vi "Práctica01_Ejercicio2_4.vi"() -> ()   [LabVIEW 2020]
panel:
  out "?":string
  in  "Selector de Operación":i16(knob) scale=0.0..3.0
  in  "y":dbl
  in  "x":dbl
  # "Resta"
  # "Multiplicacion"
  # "Division"
  # "Suma"
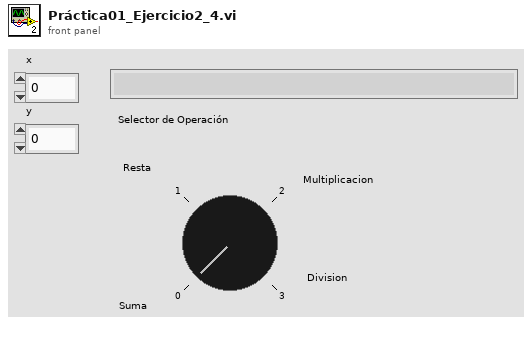
[diagram p1: front panel]
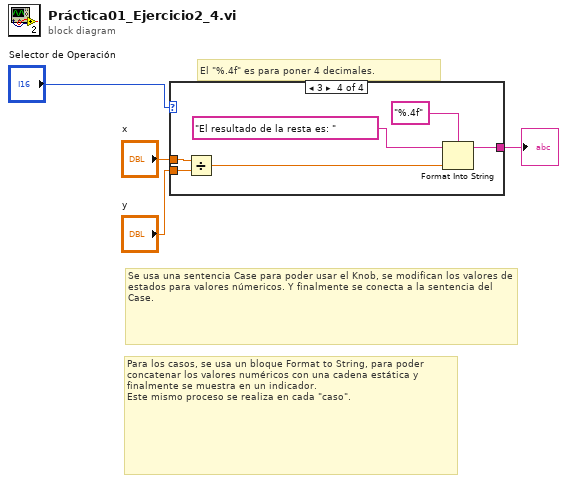
[diagram p0: block diagram]
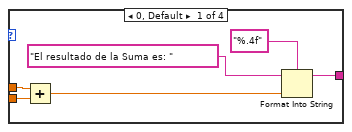
[diagram p2: hidden frame]
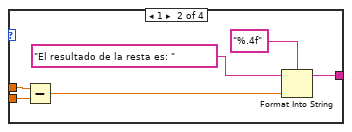
[diagram p3: hidden frame]
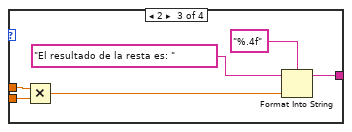
[diagram p4: hidden frame]
diagram:
  # "Para los casos, se usa un bloque Format to String, para poder concatenar los valores numéricos con una cadena estática y finalmente se muestra en un indicador.\nEste mismo proceso se realiza en cada \"caso\"."
  # "Se usa una sentencia Case para poder usar el Knob, se modifican los valores de estados para valores númericos. Y finalmente se conecta a la sentencia del Case."
  # "El \"%.4f\" es para poner 4 decimales."
  n1 = case shown="3" "Selector de Operación" {
    tunnel: [w5 w12 w17 w23] -> w3
    tunnel: "x" -> [w10 w16 w19 w25]
    tunnel: "y" -> [w9 w15 w18 w24]
    frame 0, Default {
      n2 = Add(x=w10, y=w9) -> (x+y=w6:dbl)
      n3 = Format Into String(format string="%.4f", initial string="El resultado de la Suma es: ", w6) -> (resulting string=w5:string)  [unwired: 1 in, 1 out]
    }
    frame 1 {
      n4 = Subtract(x=w16, y=w15) -> (x-y=w13:dbl)
      n5 = Format Into String(format string="%.4f", initial string="El resultado de la resta es: " ("string"), w13) -> (resulting string=w12:string)  [unwired: 1 in, 1 out]
    }
    frame 2 {
      n6 = Multiply(x=w19, y=w18) -> (x*y=w20:dbl)
      n7 = Format Into String(format string="%.4f", initial string="El resultado de la resta es: " ("string"), w20) -> (resulting string=w17:string)  [unwired: 1 in, 1 out]
    }
    frame 3 {
      n8 = Divide(x=w25, y=w24) -> (x/y=w26:dbl)
      n9 = Format Into String(format string="%.4f", initial string="El resultado de la resta es: " ("string"), w26) -> (resulting string=w23:string)  [unwired: 1 in, 1 out]
    }
  }
  "?" <- w3
